vi "Kelvinox_Merge_Cluster.vi"(1 "Kelvinox-Control":T3, 2 "Kelvinox-Status":T2 {"Sorb Heater" format="%#.0f"; "Still Heater" format="%#.0f"; "MC Heater" format="%#.0f"; "Sample" format="%_3g"; "4K" format="%_3g"; "MC" format="%_3g"; "Cold\nPlate" format="%_3g"; "1K Pot" format="%_3g"; "Still" format="%_3g"; "P5" format="%_3f"; "P4" format="%_3f"; "P3" format="%_3f"; "P2" format="%_3f"; "P1" format="%_3g"; "Dump" scale=0.0..755.0}) -> (0 "Kelvinox-Cluster":T1 {"Sorb" format="%_3g"; "MC Heater" format="%#.0f"; "Sorb Heater" format="%#.0f"; "Still Heater" format="%#.0f"; "Rate (K/min)" min=0.0 max=1.0 step=0.001 format="%.3g"; "Setpoint-Manual" min=0.0 max=10.0 step=0.001 format="%.3f"; "T-Setpoint" format="%.3f"; "Sample" format="%_3g"; "4K" format="%_3g"; "MC" format="%_3g"; "Cold\nPlate" format="%_3g"; "1K Pot" format="%_3g"; "Still" format="%_3g"; "P5" format="%_3f"; "P4" format="%_3f"; "P3" format="%_3f"; "P2" format="%_3f"; "P1" format="%_3g"; "Dump" scale=0.0..1000.0})   [LabVIEW 2019]
uses:
  Kelvinox/Kelvinox_Control.ctl
  Kelvinox/Kelvinox_Status.ctl
  Kelvinox/Kelvinox_Cluster.ctl
panel:
  # "Hz"
  # "Pressures in mbar"
  # "Temperatures in K"
  # "Heater Outputs\nin µW"
  # "DU"
  # "He\nTrap"
  # "LN2\nTrap"
  # "Hz"
  # "Pressures in mbar"
  # "Temperatures in K"
  # "Heater Outputs in µW"
  # "DU"
  # "He\nTrap"
  # "LN2\nTrap"
  # "Pressures in mbar"
  # "Temperatures in K"
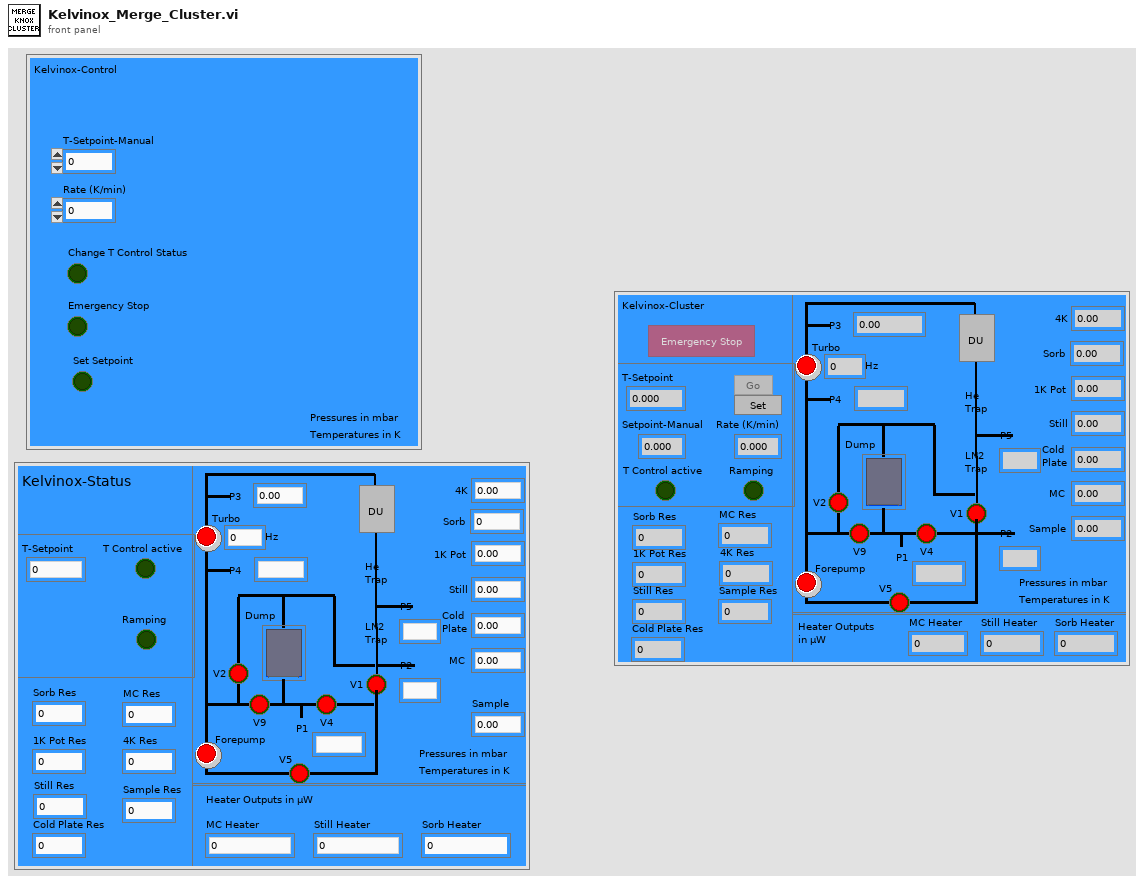
[diagram p1: front panel]
types:
  T1 = typedef "Kelvinox_Cluster.ctl" = cluster{"V1":bool, "V2":bool, "Dump":u16, "V4":bool, "V5":bool, "V9":bool, "P1":dbl, "P2":dbl, "P3":dbl, "P4":dbl, "P5":dbl, "Turbo":bool, "Forepump":bool, "speed":dbl, "Sorb":dbl, "1K Pot":dbl, "Still":dbl, "Cold\nPlate":dbl, "MC":dbl, "4K":dbl, "Sample":dbl, "T-Setpoint":dbl, "Setpoint-Manual":dbl, "Rate (K/min)":dbl, "Emergency Stop":bool, "Still Heater":dbl, "Sorb Heater":dbl, "T Control active":bool, "MC Heater":dbl, "Sorb Res":dbl, "1K Pot Res":dbl, "Still Res":dbl, "Cold Plate Res":dbl, "MC Res":dbl, "4K Res":dbl, "Sample Res":dbl, "Set Setpoint":bool, "Ramping":bool, "Change T Control Status":bool}
  T2 = typedef "Kelvinox_Status.ctl" = cluster{"V1":bool, "V2":bool, "Dump":u16, "V4":bool, "V5":bool, "V9":bool, "P1":dbl, "P2":dbl, "P3":dbl, "P4":dbl, "P5":dbl, "Turbo":bool, "Forepump":bool, "speed":dbl, "Sorb":dbl, "1K Pot":dbl, "Still":dbl, "Cold\nPlate":dbl, "MC":dbl, "4K":dbl, "Sample":dbl, "T-Setpoint":dbl, "MC Heater":dbl, "Still Heater":dbl, "Sorb Heater":dbl, "T Control active":bool, "Sorb Res":dbl, "1K Pot Res":dbl, "Still Res":dbl, "Cold Plate Res":dbl, "MC Res":dbl, "4K Res":dbl, "Sample Res":dbl, "Ramping":bool}
  T3 = typedef "Kelvinox_Control.ctl" = cluster{"T-Setpoint-Manual":dbl, "Rate (K/min)":dbl, "Change T Control Status":bool, "Emergency Stop":bool, "Set Setpoint":bool}
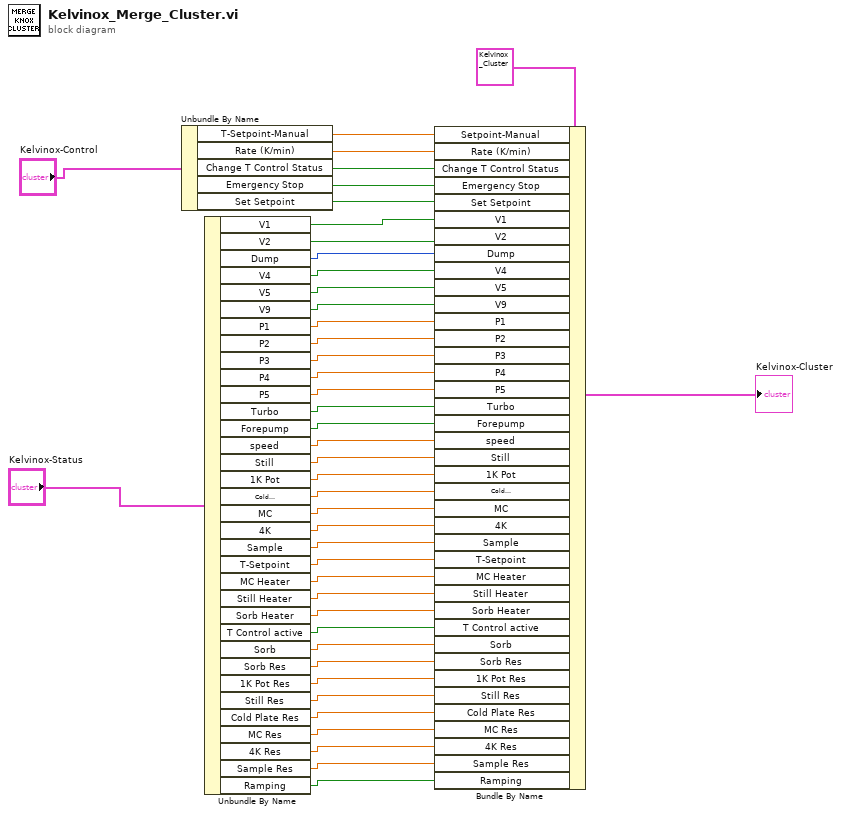
[diagram p0: block diagram]
diagram:
  n1 = Unbundle By Name("Kelvinox-Control") -> ("T-Setpoint-Manual"=w40:dbl, "Rate (K/min)"=w39:dbl, "Change T Control Status"=w38:bool, "Emergency Stop"=w37:bool, "Set Setpoint"=w2:bool)
  n2 = Unbundle By Name("Kelvinox-Status") -> ("V1"=w36:bool, "V2"=w35:bool, "Dump"=w34:u16, "V4"=w33:bool, "V5"=w32:bool, "V9"=w31:bool, "P1"=w30:dbl, "P2"=w29:dbl, "P3"=w28:dbl, "P4"=w27:dbl, "P5"=w26:dbl, "Turbo"=w24:bool, "Forepump"=w23:bool, "speed"=w22:dbl, "Still"=w21:dbl, "1K Pot"=w20:dbl, "Cold\nPlate"=w19:dbl, "MC"=w18:dbl, "4K"=w17:dbl, "Sample"=w16:dbl, "T-Setpoint"=w15:dbl, "MC Heater"=w14:dbl, "Still Heater"=w13:dbl, "Sorb Heater"=w12:dbl, "T Control active"=w11:bool, "Sorb"=w10:dbl, "Sorb Res"=w9:dbl, "1K Pot Res"=w8:dbl, "Still Res"=w7:dbl, "Cold Plate Res"=w6:dbl, "MC Res"=w5:dbl, "4K Res"=w4:dbl, "Sample Res"=w3:dbl, "Ramping"=w1:bool)
  n3 = Bundle By Name(cluster=T1 {"V1"=FALSE, "V2"=FALSE, "Dump"=0, "V4"=FALSE, "V5"=FALSE, "V9"=FALSE, "P1"=0.0, "P2"=0.0, "P3"=0.0, "P4"=0.0, "P5"=0.0, "Turbo"=FALSE, "Forepump"=FALSE, "speed"=0.0, "Sorb"=0.0, "1K Pot"=0.0, "Still"=0.0, "Cold\nPlate"=0.0, "MC"=0.0, "4K"=0.0, "Sample"=0.0, "T-Setpoint"=0.0, "Setpoint-Manual"=0.0, "Rate (K/min)"=0.0, "Emergency Stop"=FALSE, "Still Heater"=0.0, "Sorb Heater"=0.0, "T Control active"=FALSE, "MC Heater"=0.0, "Sorb Res"=0.0, "1K Pot Res"=0.0, "Still Res"=0.0, "Cold Plate Res"=0.0, "MC Res"=0.0, "4K Res"=0.0, "Sample Res"=0.0, "Set Setpoint"=FALSE, "Ramping"=FALSE, "Change T Control Status"=FALSE} ("Kelvinox-Cluster"), "Setpoint-Manual"=w40, "Rate (K/min)"=w39, "Change T Control Status"=w38, "Emergency Stop"=w37, "Set Setpoint"=w2, "V1"=w36, "V2"=w35, "Dump"=w34, "V4"=w33, "V5"=w32, "V9"=w31, "P1"=w30, "P2"=w29, "P3"=w28, "P4"=w27, "P5"=w26, "Turbo"=w24, "Forepump"=w23, "speed"=w22, "Still"=w21, "1K Pot"=w20, "Cold\nPlate"=w19, "MC"=w18, "4K"=w17, "Sample"=w16, "T-Setpoint"=w15, "MC Heater"=w14, "Still Heater"=w13, "Sorb Heater"=w12, "T Control active"=w11, "Sorb"=w10, "Sorb Res"=w9, "1K Pot Res"=w8, "Still Res"=w7, "Cold Plate Res"=w6, "MC Res"=w5, "4K Res"=w4, "Sample Res"=w3, "Ramping"=w1) -> (→"Kelvinox-Cluster":T1)
